vi "Dequeue all Coinchunt Results.vi"(8 "error in (no error)":errorcluster, 11 "Queue in":refnum<queue>) -> (0 "error out":errorcluster, 1 "elements dequeued":i32, 2 "Dequeued elements":T1[](array[typedef]), 3 "Queue out":refnum<queue>)   [LabVIEW 2016]
uses:
  Typedefs/Primary channel coincidence hunt.ctl
  Typedefs/Coincidence.ctl
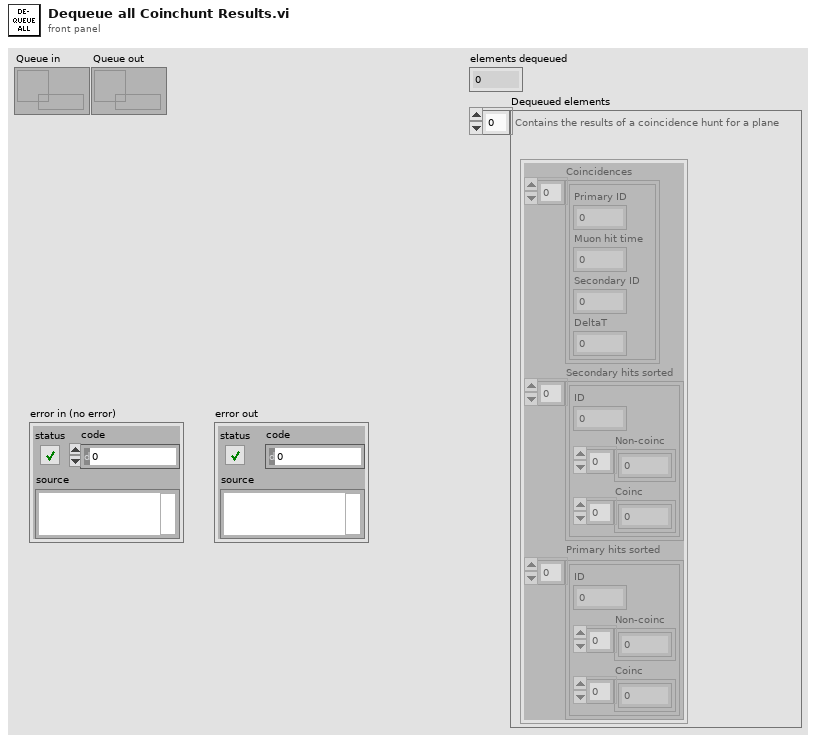
[diagram p1: front panel]
types:
  T1 = typedef "Primary channel coincidence hunt.ctl" = cluster{"Coincidences":T2[], "Secondary hits sorted":cluster{"ID":i8, "Non-coinc":u64[], "Coinc":u64[]}[], "Primary hits sorted":cluster{"ID":i8, "Non-coinc":u64[], "Coinc":u64[]}[]}
  T2 = typedef "Coincidence.ctl" = cluster{"Primary ID":i8, "Muon hit time":u64, "Secondary ID":i8, "DeltaT":i32}
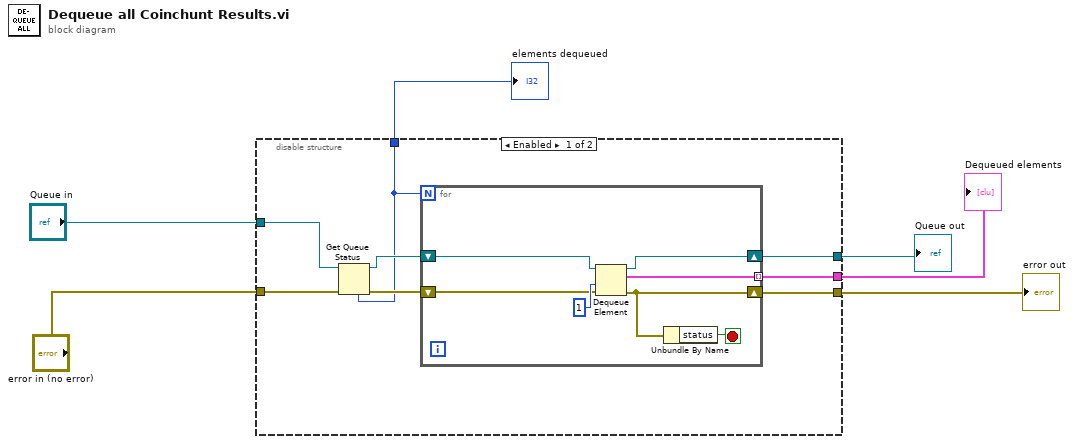
[diagram p0: block diagram]
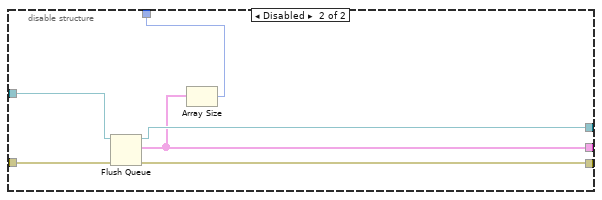
[diagram p2: hidden frame]
diagram:
  n1 = disable-structure shown="Enabled" {
    disable-tunnel: [w14 w24] -> w3
    disable-tunnel: "error in (no error)" -> [w13 w27]
    disable-tunnel: [w10 w22] -> w5
    disable-tunnel: "Queue in" -> [w9 w26]
    disable-tunnel: [w8 w25] -> w2
    disable-tunnel: [w7 w23] -> w1
    frame Enabled {
      n2 = Get Queue Status(queue=w9, error in (no error)=w13) -> (queue out=w11:refnum<queue>, error out=w12:errorcluster, # elements in queue=w10:i32)  [unwired: 1 in, 5 out]
      n3 = for {
        N: w10 -> [_]
        shift-right: [w20] -> w14
        shift-left: w12 -> [w18]
        shift-right: [w21] -> w8
        shift-left: w11 -> [w17]
        tunnel: [w15] -> w7 mode=indexing
        stop <- w16 stop-if-true
        n4 = Dequeue Element(queue=w17, timeout in ms (-1)=1, error in (no error)=w18) -> (queue out=w21:refnum<queue>, element=w15:T1, error out=w20:errorcluster)  [unwired: 1 out]
        n5 = Unbundle By Name(w20) -> ("status"=w16:bool)
      }
    }
    frame Disabled {
      n6 = Flush Queue(queue=w26, error in (no error)=w27) -> (queue out=w25:refnum<queue>, remaining elements=w23:T1[], error out=w24:errorcluster)
      n7 = Array Size(array=w23) -> (size(s)=w22:i32)
    }
  }
  "elements dequeued" <- w5
  "error out" <- w3
  "Queue out" <- w2
  "Dequeued elements" <- w1
